vi "Check Persistent Decorator Actors.vi"(10 "Persistent Decorator Actors":refnum<class "Actor.lvclass">[](array[class])) -> (2 "Error":errorcluster)   [LabVIEW 2025, in "jettl.lvlib"]
uses:
  jettl.lvlib
  Actor/Actor.lvclass
  Error/Error.lvlib
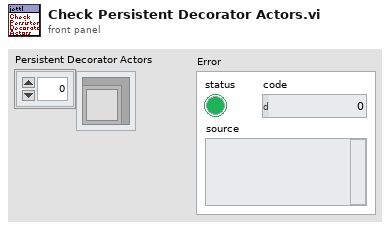
[diagram p1: front panel]
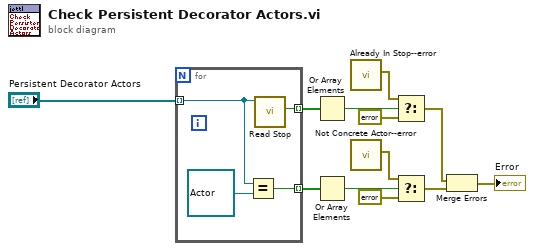
[diagram p0: block diagram]
diagram:
  n1 = for {
    tunnel: "Persistent Decorator Actors" -> [w14] mode=indexing
    tunnel: [w16] -> w1 mode=indexing
    tunnel: [w13] -> w2 mode=indexing
    n2 = Equal?(x=w14, y=refnum<class "Actor.lvclass"> refnum ("jettl.lvlib:Actor.lvclass")) -> (x = y?=w13:bool)
    n3 = call-dynamic "Read Stop.vi"("Actor in"=w14) -> ("Stop"=w16:bool)  [unwired: 10 in]
  }
  n4 = Or Array Elements(Boolean array=w1) -> (logical OR=w7:bool)
  n5 = Or Array Elements(Boolean array=w2) -> (logical OR=w10:bool)
  n6 = call "Already In Stop--error.vi"() -> ("Error"=w8:errorcluster)  [unwired: 11 in]
  n7 = call "Not Concrete Actor--error.vi"() -> ("Error"=w11:errorcluster)  [unwired: 11 in]
  n8 = Select(t=w8, s=w7, f=errorcluster {"status"=FALSE, "code"=0, "source"=""}) -> (s? t:f=w3:errorcluster)
  n9 = Select(t=w11, s=w10, f=errorcluster {"status"=FALSE, "code"=0, "source"=""}) -> (s? t:f=w4:errorcluster)
  n10 = Merge Errors(w3, w4) -> (→"Error":errorcluster)
